vi "Test Caller.vi"(8 "error in (no error)":errorcluster, 10 "Test Symbols":T2[](array[typedef])=[{"Symbol Name"="TestVariable1", "Symbol Value"="Double"}], 11 "Test Harness":path=path "C:/Users/Natan Biesmans/Documents/Project-Bedrock/Demo Tests/Test Harness.vi") -> (0 "error out":errorcluster, 2 "Test Error Out":errorcluster, 3 "Results":T1[](array[typedef]), 4 "UI Inidicators Values":cluster{"Name":string, "Variant Data":variant}[](array[cluster]))   [LabVIEW 2020]
uses:
  Test Symbol.ctl
  Test Results.ctl
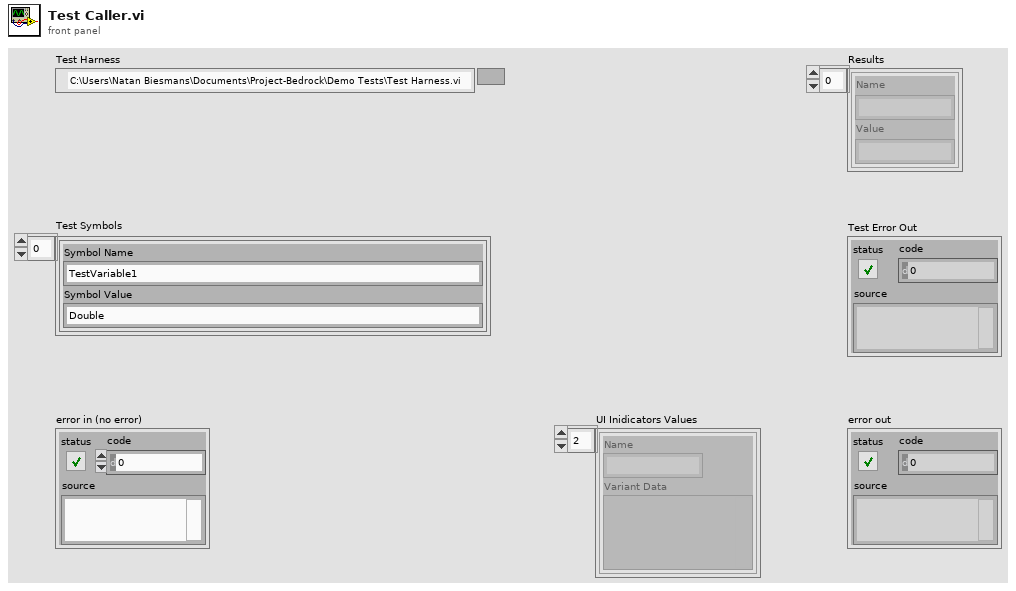
[diagram p1: front panel]
types:
  T1 = typedef "Test Results.ctl" = cluster{"Name":string, "Value":string}
  T2 = typedef "Test Symbol.ctl" = cluster{"Symbol Name":string, "Symbol Value":string}
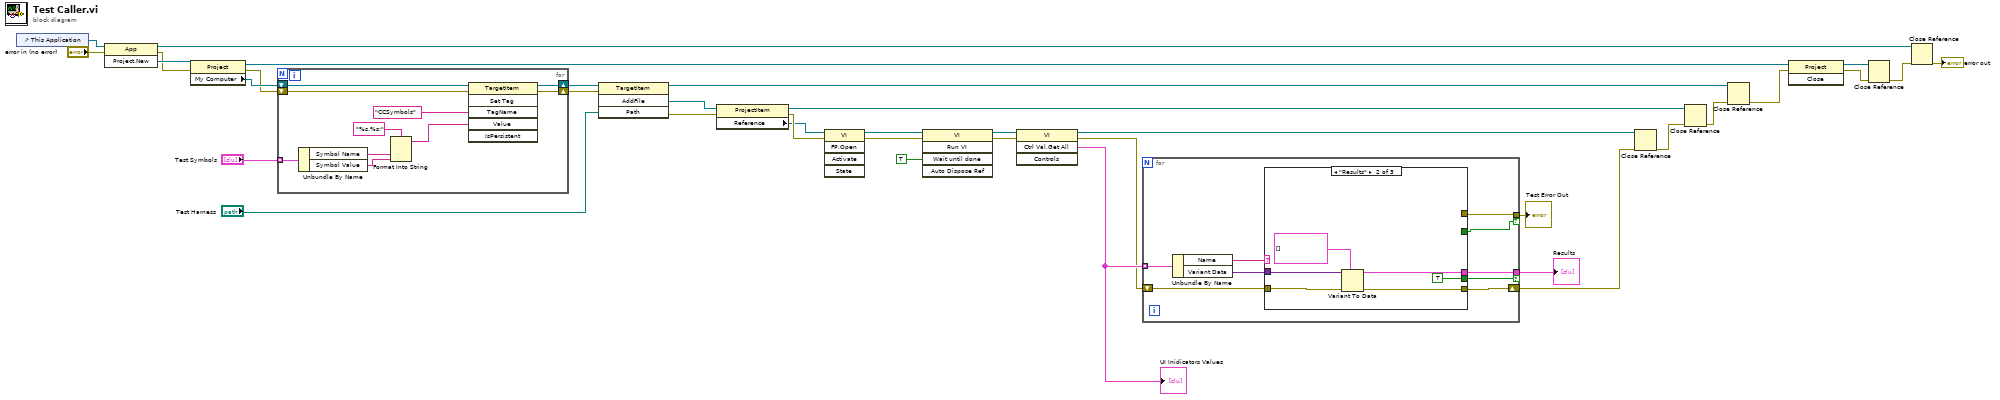
[diagram p0: block diagram]
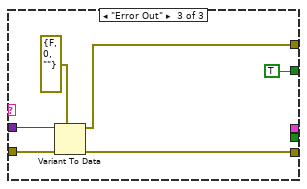
[diagram p3: hidden frame]
diagram:
  n1 = control-ref of="This Application"() -> (w36:refnum<vi>)
  n2 = invoke class="App" method="Project.New"(reference=w36, error in="error in (no error)") -> (reference out=w29:refnum<vi>, error out=w34:errorcluster, "Project:New"=w35:refnum<vi>)  [unwired: 1 in]
  n3 = property class="Project"(reference=w35, error in=w34) -> (reference out=w8:refnum<vi>, error out=w25:errorcluster, "My Computer"=w27:refnum<vi>)
  n4 = for {
    shift-right: [w45] -> w26
    shift-left: w27 -> [w46]
    shift-right: [w43] -> w24
    shift-left: w25 -> [w44]
    tunnel: "Test Symbols" -> [w39] mode=indexing
    n5 = Unbundle By Name(w39) -> ("Symbol Name"=w38:string, "Symbol Value"=w37:string)
    n6 = Format Into String(format string="%s,%s;", w38, w37) -> (resulting string=w40:string)  [unwired: 2 in, 1 out]
    n7 = invoke class="TargetItem" method="Set Tag"(reference=w46, error in=w44, "TagName"="CCSymbols" ("Tag Name"), "Value"=w40) -> (reference out=w45:refnum<vi>, error out=w43:errorcluster)  [unwired: 2 in, 4 out]
  }
  n8 = invoke class="TargetItem" method="AddFile"(reference=w26, error in=w24, "Path"="Test Harness") -> (reference out=w33:refnum<vi>, error out=w28:errorcluster, "AddFile"=w31:refnum<vi>)  [unwired: 1 in, 1 out]
  n9 = property class="ProjectItem"(reference=w31, error in=w28) -> (reference out=w20:refnum<vi>, error out=w4:errorcluster, "Reference"=w3:refnum<vi>)
  n10 = invoke class="VI" method="FP.Open"(reference=w3, error in=w4) -> (reference out=w2:refnum<vi>, error out=w1:errorcluster)  [unwired: 3 in, 3 out]
  n11 = invoke class="VI" method="Run VI"(reference=w2, error in=w1, "Wait until done"=TRUE ("Wait Until Done")) -> (reference out=w16:refnum<vi>, error out=w15:errorcluster)  [unwired: 2 in, 3 out]
  n12 = invoke class="VI" method="Ctrl Val.Get All"(reference=w16, error in=w15) -> (reference out=w14:refnum<vi>, error out=w12:errorcluster, "Get All Control Values Variant"=w13:cluster{"Name":string, "Variant Data":variant}[])  [unwired: 2 in, 1 out]
  "UI Inidicators Values" <- w13
  n13 = for {
    tunnel: w13 -> [w55] mode=indexing
    shift-right: [w51] -> w11
    shift-left: w12 -> [w52]
    tunnel: [w50] -> w10 if=w49
    tunnel: [w48] -> w9 if=w47
    n14 = Unbundle By Name(w55) -> ("Name"=w54:string, "Variant Data"=w53:variant)
    n15 = case shown="\"Results\"" w54 {
      tunnel: w53 -> [_ w62 w67]
      tunnel: w52 -> [w56 w61 w68]
      tunnel: [w56 w60 w64] -> w51
      tunnel: [_ w59 _] -> w50
      tunnel: [_ TRUE _] -> w49
      tunnel: [_ _ w65] -> w48
      tunnel: [_ _ TRUE] -> w47
      frame Default {
      }
      frame "Results" {
        n16 = Variant To Data(error in=w61, type=T1[] [], Variant=w62) -> (data=w59:T1[], error out=w60:errorcluster)
      }
      frame "Error Out" {
        n17 = Variant To Data(error in=w68, type=errorcluster {"status"=FALSE, "code"=0, "source"=""} ("error constant"), Variant=w67) -> (data=w65:errorcluster, error out=w64:errorcluster)
      }
    }
  }
  "Results" <- w10
  "Test Error Out" <- w9
  n18 = Close Reference(reference=w14, error in (no error)=w11) -> (error out=w22:errorcluster)
  n19 = Close Reference(reference=w20, error in (no error)=w22) -> (error out=w21:errorcluster)
  n20 = Close Reference(reference=w33, error in (no error)=w21) -> (error out=w7:errorcluster)
  n21 = invoke class="Project" method="Close"(reference=w8, error in=w7) -> (reference out=w6:refnum<vi>, error out=w5:errorcluster)  [unwired: 1 in, 1 out]
  n22 = Close Reference(reference=w6, error in (no error)=w5) -> (error out=w32:errorcluster)
  n23 = Close Reference(reference=w29, error in (no error)=w32) -> (error out=→"error out":errorcluster)
